vi "Is Open For Edit.vi"(8 "error in (no error)":errorcluster, 11 "Tree in":refnum<class "Tree.lvclass">) -> (0 "error out":errorcluster, 2 "Is open for edit?":bool, 3 "Tree out":refnum<class "Tree.lvclass">)   [LabVIEW 2013, in "MDSplus.lvlib" / "Tree.lvclass"]
uses:
  <vilib>/MDSplus/Classes/Tree_Class/Tree.lvclass
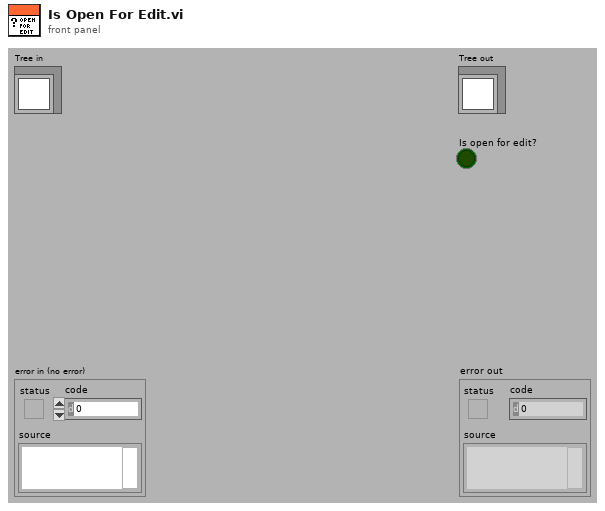
[diagram p1: front panel]
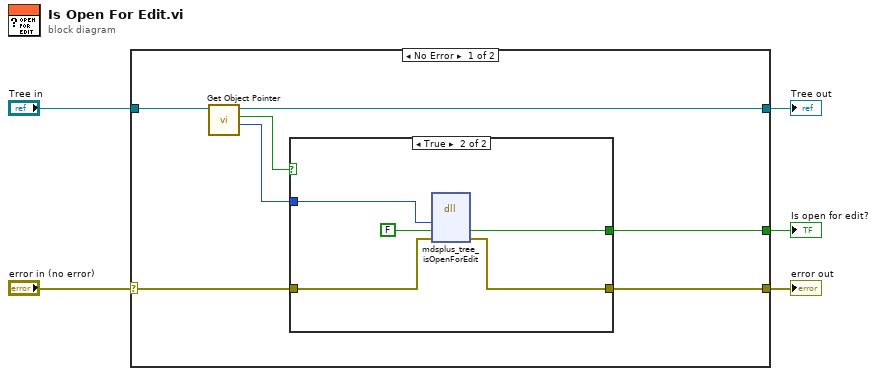
[diagram p0: block diagram]
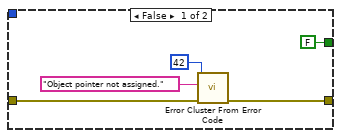
[diagram p2: hidden frame]
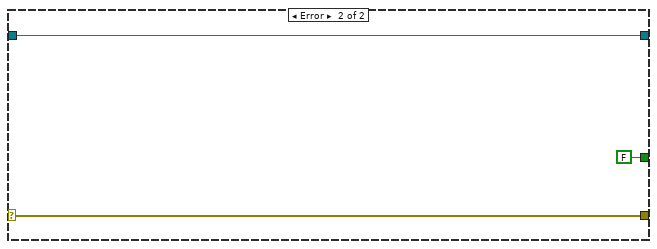
[diagram p3: hidden frame]
diagram:
  n1 = case shown="No Error" "error in (no error)" {
    selector: "error in (no error)" -> [w7 w25]
    tunnel: [w6 w25] -> w4
    tunnel: [w10 w24] -> w2
    tunnel: "Tree in" -> [w11 w24]
    tunnel: [w12 FALSE] -> w1
    frame No Error {
      n2 = call-dynamic "Get Object Pointer.vi"("Tree in"=w11) -> ("Object Pointer"=w8:i64, "Assigned object pointer?"=w9:bool, "Tree out"=w10:refnum<class "Tree.lvclass">)  [unwired: 8 in]
      n3 = case shown="True" w9 {
        tunnel: [FALSE w22] -> w12
        tunnel: w8 -> [_ w21]
        tunnel: w7 -> [w15 w20]
        tunnel: [w14 w19] -> w6
        frame False {
          n4 = call <vilib>:"Error Cluster From Error Code.vi"("error in (no error)"=w15, "error message (\"\")"="Object pointer not assigned." ("error message (\"\")"), "error code (0)"=42) -> ("error out"=w14:errorcluster)  [unwired: 6 in]
        }
        frame True {
          n5 = dll-call lib="MDSobjectsLVShr" fn="mdsplus_tree_isOpenForEdit"("lvTreePtr"=w21, "lvIsOpenForEditOut"=FALSE, "error"=w20) -> ("lvIsOpenForEditOut"=w22:bool, "error"=w19:errorcluster)  [unwired: 5 in, 2 out]
        }
      }
    }
    frame Error {
    }
  }
  "error out" <- w4
  "Tree out" <- w2
  "Is open for edit?" <- w1
